vi "Remove from 2D array Str.vi"(10 "Characters to Remove":string[](array[string])=["\n", "\t"], 11 "Strings In":string[][](array[string])) -> (3 "Result Strings Out":string[][](array[string]))   [LabVIEW 2018, in "Vires VTD System Explorer.lvlib"]
uses:
  Vires VTD System Explorer.lvlib
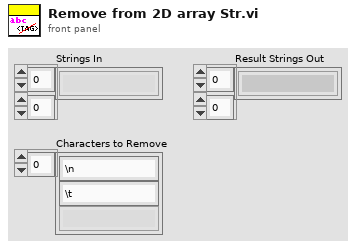
[diagram p1: front panel]
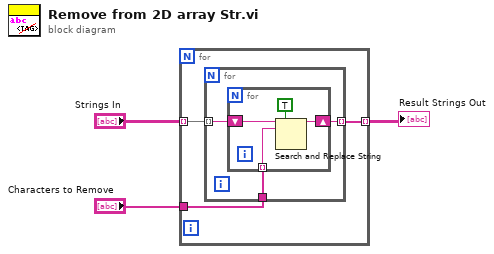
[diagram p0: block diagram]
diagram:
  n1 = for {
    tunnel: "Strings In" -> [w5] mode=indexing
    tunnel: [w6] -> w1 mode=indexing
    tunnel: "Characters to Remove" -> [w4]
    n2 = for {
      tunnel: [w8] -> w6 mode=indexing
      tunnel: w5 -> [w9] mode=indexing
      tunnel: w4 -> [w7]
      n3 = for {
        shift-right: [w12] -> w8
        shift-left: w9 -> [w13]
        tunnel: w7 -> [w10] mode=indexing
        n4 = Search and Replace String(replace all?=TRUE ("replace all? (F)"), input string=w13, search string=w10) -> (result string=w12:string)  [unwired: 5 in, 3 out]
      }
    }
  }
  "Result Strings Out" <- w1
